vi "油压mA2MPa.vi"(3 "油压Max":dbl=25.0, 4 "油压mA":dbl, 5 "油压Min":dbl) -> (1 "油压MPa":dbl)   [LabVIEW 2013]
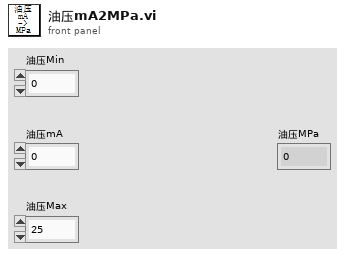
[diagram p1: front panel]
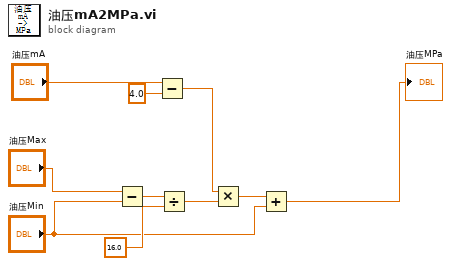
[diagram p0: block diagram]
diagram:
  n1 = Subtract(x="油压Max", y="油压Min") -> (x-y=w9:dbl)
  n2 = Subtract(x="油压mA", y=4.0) -> (x-y=w4:dbl)
  n3 = Divide(x=w9, y=16.0) -> (x/y=w7:dbl)
  n4 = Multiply(x=w4, y=w7) -> (x*y=w3:dbl)
  n5 = Add(x=w3, y="油压Min") -> (x+y=→"油压MPa":dbl)
